vi "TestPassIf.vi"(8 "error in (no error)":errorcluster, 11 "TestCase in":refnum<class "CalculatorTestCase.lvclass">) -> (0 "error out":errorcluster, 3 "TestCase out":refnum<class "CalculatorTestCase.lvclass">)   [LabVIEW 2020, in "CalculatorTestCase.lvclass"]
uses:
  CalculatorTestCase.lvclass
  LabVIEW Data/Calculator/Calculator.lvclass
  <vilib>/addons/_JKI Toolkits/VI Tester/TestCase.llb/TestCase.lvclass
  C:/Program Files (x86)/National Instruments/LabVIEW 2020/vi.lib/addons/_JKI Toolkits/VI Tester/TestCase.llb/TestCase.lvclass
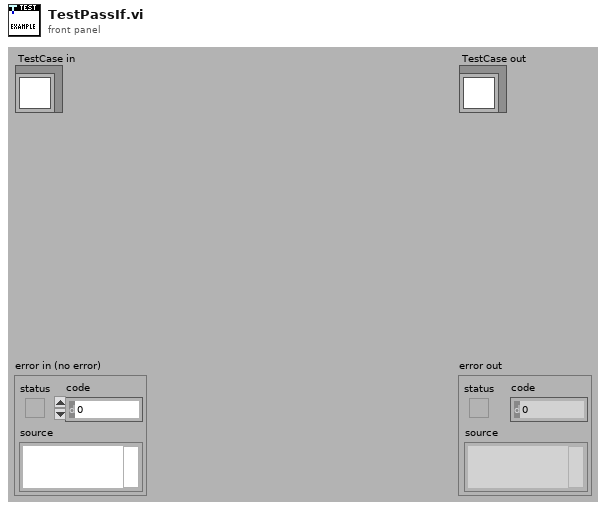
[diagram p1: front panel]
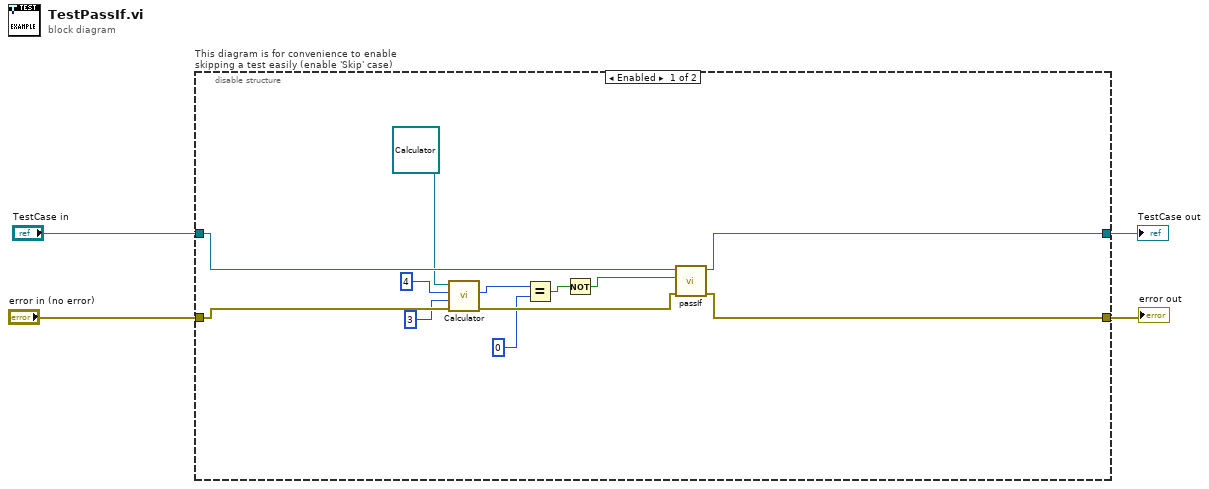
[diagram p0: block diagram]
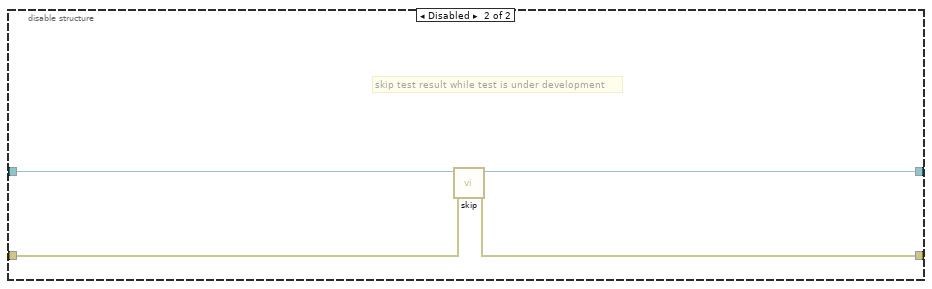
[diagram p2: hidden frame]
diagram:
  n1 = disable-structure "This diagram is for convenience to enable skipping a test easily (enable 'Skip' case)" shown="Enabled" {
    disable-tunnel: "TestCase in" -> [w16 w20]
    disable-tunnel: [w15 w18] -> w1
    disable-tunnel: [w12 w19] -> w3
    disable-tunnel: "error in (no error)" -> [w14 w17]
    frame Enabled {
      n2 = call "Calculator.vi"("error in (no error)"=w14, "Input 2"=3, "Input 1"=4, "Calculator in"=refnum<class "Calculator.lvclass"> refnum) -> ("error out"=w13:errorcluster, "Output"=w8:i32)  [unwired: 5 in, 1 out]
      n3 = Equal?(x=w8, y=0) -> (x = y?=w6:bool)
      n4 = Not(x=w6) -> (.not. x?=w5:bool)
      n5 = call-dynamic "passIf.vi"("error in (no error)"=w13, "pass"=w5, "TestCase in"=w16) -> ("error out"=w12:errorcluster, "TestCase out"=w15:refnum<class "CalculatorTestCase.lvclass">)  [unwired: 7 in]
    }
    frame Disabled {
      # "skip test result while test is under development"
      n6 = call <vilib>:"skip.vi"("error in (no error)"=w17, "TestCase in"=w20) -> ("error out"=w19:errorcluster, "TestCase out"=w18:refnum<class "CalculatorTestCase.lvclass">)  [unwired: 8 in]
    }
  }
  "error out" <- w3
  "TestCase out" <- w1
